vi "AVI-Viewer cleanup.vi"(8 "error in (no error)":errorcluster, 9 "RGB image ref":T1, 10 "I16 image ref":T1) -> (0 "error out":errorcluster)   [LabVIEW 2020]
uses:
  <vilib>/vision/Image Controls.llb/IMAQ Image.ctl
  Typedefs/Save-Load enum.ctl
  Globals/gl_Time series viewer globals.vi
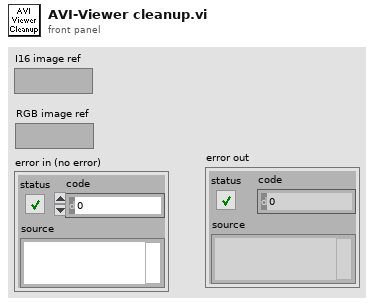
[diagram p1: front panel]
types:
  T1 = typedef "IMAQ Image.ctl" = refnum<image>
  T2 = typedef "Save-Load enum.ctl" = enum16{"Save to file", "Load from file", "Compare from file", "Save Backup"}
  T3 = enum16{"None", "Release queue", "Obtain queue", "Enqueue", "Get status", "Set status"}
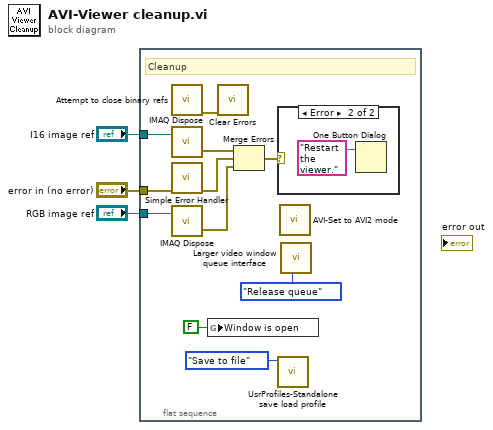
[diagram p0: block diagram]
diagram:
  n1 = flat-sequence {
    tunnel: "I16 image ref" -> [w14]
    tunnel: "error in (no error)" -> [w11]
    tunnel: "RGB image ref" -> [w9]
    frame #0 {
      # "Cleanup"
      n2 = call "Attempt to close binary refs.vi"() -> ("error out"=w5:errorcluster)  [unwired: 11 in]
      n3 = call "IMAQ Dispose"("Image"=w14) -> ("error out"=w12:errorcluster)  [unwired: 5 in]
      n4 = call <vilib>:"Simple Error Handler.vi"("error in (no error)"=w11) -> ("error out"=w10:errorcluster)  [unwired: 4 in, 4 out]
      n5 = call "IMAQ Dispose"("Image"=w9) -> ("error out"=w8:errorcluster)  [unwired: 5 in]
      n6 = global write "gl_Time series viewer globals.vi" "Window is open"(FALSE ("Window is open")) -> ()
      n7 = call <vilib>:"Clear Errors.vi"("error in (no error)"=w5) -> ()  [unwired: 5 in, 2 out]
      n8 = Merge Errors(w12, w10, w8) -> (w13:errorcluster)
      n9 = case shown="Error" w13 {
        frame No Error {
        }
        frame Error {
          n10 = One Button Dialog(message="Restart the viewer.") -> ()  [unwired: 1 in, 1 out]
        }
      }
      n11 = call "UsrProfiles-Standalone save load profile.vi"("Function"=Save-Load_enum."Save to file") -> ()  [unwired: 10 in, 1 out]
      n12 = call "AVI-Set to AVI2 mode.vi"() -> ()  [unwired: 11 in, 1 out]
      n13 = call "Larger video window queue interface.vi"("Function"=T3."Release queue") -> ()  [unwired: 10 in, 1 out]
    }
  }
